vi "List_API_Functions.vi"() -> (0 "API Functions Table":cluster{string, string, path}[](array[cluster]))   [LabVIEW 2011]
doc: "This VI scans the \"api\" directory for VI files, which are then loaded into memory so they may be called as polymorphic API VI functions."
panel:
  in  "Type Specifier":refnum<vi>
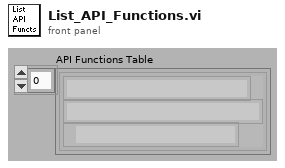
[diagram p1: front panel]
types:
  T1 = cluster{string, "Front Panel.Title":string, "appended path":path}
  T2 = cluster{string, "Front Panel.Title":string, "appended path":path}[]
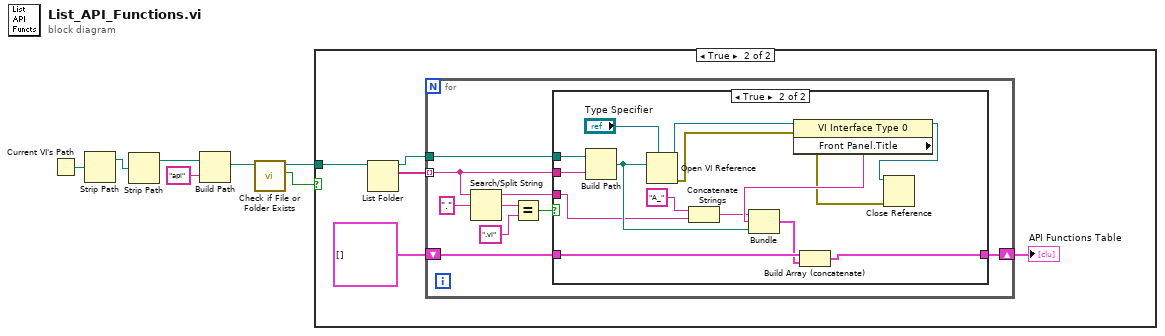
[diagram p0: block diagram]
diagram:
  n1 = Current VI's Path() -> (path=w7:path)
  n2 = Strip Path(path=w7) -> (stripped path=w5:path)  [unwired: 1 out]
  n3 = Strip Path(path=w5) -> (stripped path=w4:path)  [unwired: 1 out]
  n4 = Build Path(base path=w4, name or relative path="api") -> (appended path=w3:path)
  n5 = call <vilib>:"Check if File or Folder Exists.vi"("path"=w3) -> ("file or folder exists?"=w1:bool, "dup path"=w2:path)  [unwired: 8 in, 1 out]
  n6 = case shown="True" w1 {
    tunnel: w2 -> [_ w8]
    frame False {
    }
    frame True {
      n7 = List Folder(path=w8) -> (path out=w11:path, filenames=w12:string[])  [unwired: 1 in, 4 out]
      n8 = for {
        tunnel: w12 -> [w20] mode=indexing
        tunnel: w11 -> [w21]
        shift-right: [w13] -> w9
        shift-left: cluster{string, string, path}[] [] -> [w14]
        n9 = Search/Split String(string=w20, search string/char (-)=".") -> (substring before match=w15:string, match + rest of string=w18:string)  [unwired: 2 out]
        n10 = Equal?(x=w18, y=".vi") -> (x = y?=w16:bool)
        n11 = case shown="True" w16 {
          tunnel: w21 -> [_ w37]
          tunnel: w20 -> [_ w36]
          tunnel: w15 -> [_ w27]
          tunnel: w14 -> [w22 w31]
          tunnel: [w22 w29] -> w13
          frame False {
          }
          frame True {
            n12 = Build Path(base path=w37, name or relative path=w36) -> (appended path=w32:path)
            n13 = Open VI Reference(type specifier VI Refnum (for type only)="Type Specifier", vi path=w32) -> (vi reference=w33:refnum<vi>, error out=w34:errorcluster)  [unwired: 2 in, 2 out]
            n14 = Concatenate Strings("A_" ("string"), w27) -> (w25:string)
            n15 = property class="VI Interface Type 0"(reference=w33, error in=w34) -> (reference out=w23:refnum<vi>, error out=w24:errorcluster, "Front Panel.Title"=w28:string)
            n16 = Bundle(w25, "Front Panel.Title"=w28, "appended path"=w32) -> (w30:T1)  [unwired: 1 out]
            n17 = Build Array (concatenate)(w31, w30) -> (w29:T2)
            n18 = Close Reference(reference=w23, error in (no error)=w24) -> ()  [unwired: 1 out]
          }
        }
      }
      "API Functions Table" <- w9
    }
  }
